vi "PV OnTool General operating info.vi"(0 "VISA session":refnum<visa-resource-name>, 5 "Adress of unit":u16=1 min=1 max=999 step=1, 7 "Parameter":u16(ring) items=[" Final rotation speed BkP [Hz]", " Motor current BkP [A]", " Motor voltage BkP [V]", " Motor power BkP [W]", " Operating hours BkP [h]", " Over temperature Controller (read only)", " Over temperature BkP (read only)"], 11 "error in (no error)":errorcluster) -> (4 "dup VISA session":refnum<visa-resource-name>, 6 "response (data)":string, 15 "error out":errorcluster)   [LabVIEW 2016, in "Pfeiffer Vacuum.lvlib"]
doc: "There are seven parameters available, only one of which can be enabled at a time. \n\n0 - Final rotations speed BkP [Hz] (default) (Para.315)\n1 - Motor current BkP [A] (Para.310)\n2 - Motor voltage BkP [V] (Para.313)\n3 - Motor power BkP [W] (Para.316)\n4 - Operating hours BkP [h] (Para.311)\n5 - Over temperature Controller (read only) (Para.304)\n6 - Over temperature BkP (read only) (Para.305)\n\nNote: read only VI"
uses:
  Pfeiffer Vacuum.lvlib
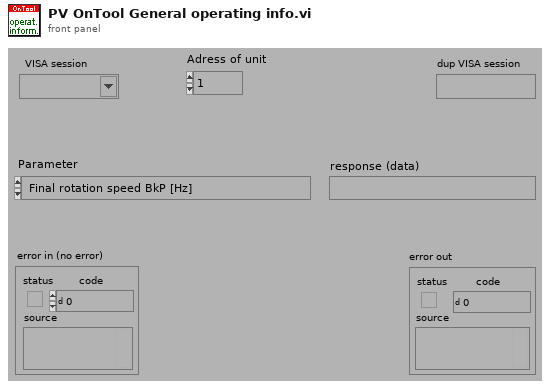
[diagram p1: front panel]
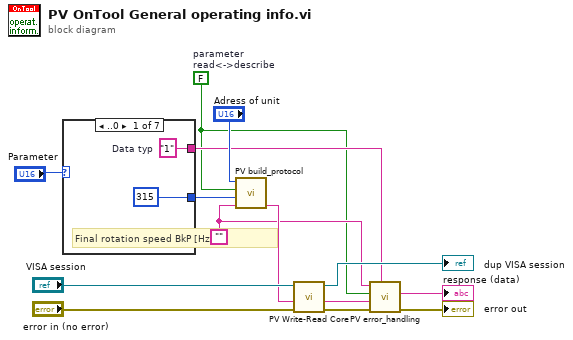
[diagram p0: block diagram]
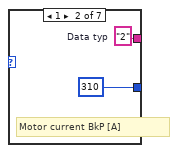
[diagram p2: hidden frame]
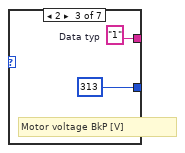
[diagram p3: hidden frame]
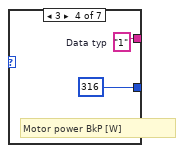
[diagram p4: hidden frame]
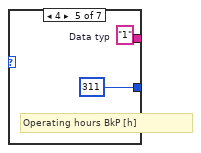
[diagram p5: hidden frame]
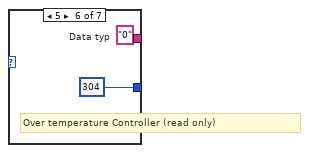
[diagram p6: hidden frame]
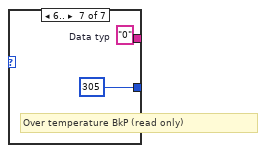
[diagram p7: hidden frame]
diagram:
  w4 = ""
  w3 = FALSE  # parameter read<->describe
  n1 = case shown="..0" "Parameter" {
    tunnel: [u16 315 ("Parameter-number") u16 310 ("Parameter-number") u16 313 ("Parameter-number") u16 316 ("Parameter-number") u16 311 ("Parameter-number") u16 304 ("Parameter-number") u16 305 ("Parameter-number")] -> w12
    tunnel: [w15 w17 w19 w21 w23 w25 w27] -> w5
    frame ..0 {
      w15 = "1"  # Data typ
      # "Final rotation speed BkP [Hz]"
    }
    frame 1 {
      w17 = "2"  # Data typ
      # "Motor current BkP [A]"
    }
    frame 2 {
      w19 = "1"  # Data typ
      # "Motor voltage BkP [V]"
    }
    frame 3 {
      w21 = "1"  # Data typ
      # "Motor power BkP [W]"
    }
    frame 4 {
      w23 = "1"  # Data typ
      # "Operating hours BkP [h]"
    }
    frame 5 {
      w25 = "0"  # Data typ
      # "Over temperature Controller (read only)"
    }
    frame 6.. {
      w27 = "0"  # Data typ
      # "Over temperature BkP (read only)"
    }
  }
  n2 = call "PV build_protocol.vi"("Data"=w4, "Parameter-number"=w12, "parameter\nread<->describe"=w3, "Adress"="Adress of unit") -> ("output"=w9:string)  [unwired: 3 in]
  n3 = call "PV Write-Read Core.vi"("error in"="error in (no error)", "Write data in"=w9, "VISA session"="VISA session") -> ("error out"=w6:errorcluster, "response (data) out"=w7:string, "dup VISA session"=→"dup VISA session":refnum<visa-resource-name>)  [unwired: 2 in]
  n4 = call "PV error_handling.vi"("Data Typ in"=w5, "error in"=w6, "response (data) in"=w7, "Parameter\nread only<->describe"=w3, "data in"=w4) -> ("error out"=→"error out":errorcluster, "Data out"=→"response (data)":string)  [unwired: 4 in, 1 out]
